vi "export.vi"(9 "Ruta luz":path, 10 "Ruta Temp":path, 11 "Curva de Luz y Temperatura 3":cluster{"Ramp Pattern":dbl[], u32[]}[](graph)=[{"Ramp Pattern"=[0.0, 0.25, 0.5, 0.75, 1.0, 1.25, 1.5, 1.75, 2.0, 2.25, 2.5, 2.75, 3.0, 3.25, 3.5, 3.75, 4.0, 4.25, 4.5, 4.75, 5.0, 5.25, 5.5, 5.75, 6.0, 6.25, 6.5, 6.75, 7.0, 7.25, 7.5, 7.75, 8.0, 8.25, 8.5, 8.75, 9.0, 9.25, 9.5, 9.75, 10.0, 10.25, 10.5, 10.75, 11.0, 11.25, 11.5, 11.75, 12.0, 12.25, 12.5, 12.75, 13.0, 13.25, 13.5, 13.75, 14.0, 14.25, 14.5, 14.75, 15.0, 15.25, 15.5, 15.75, 16.0, 16.25, 16.5, 16.75, 17.0, 17.25, 17.5, 17.75, 18.0, 18.25, 18.5, 18.75, 19.0, 19.25, 19.5, 19.75, 20.0, 20.25, 20.5, 20.75, 21.0, 21.25, 21.5, 21.75, 22.0, 22.25, 22.5, 22.75, 23.0, 23.25, 23.5, 23.75, 24.0, 24.25, 24.5, 24.75, 25.0, 25.25, 25.5, 25.75, 26.0, 26.25, 26.5, 26.75, 27.0, 27.25, 27.5, 27.75, 28.0, 28.25, 28.5, 28.75, 29.0, 29.25, 29.5, 29.75, 30.0, 30.25, 30.5, 30.75, 31.0, 31.25, 31.5, 31.75, 32.0, 32.25, 32.5, 32.75, 33.0, 33.25, 33.5, 33.75, 34.0, 34.25, 34.5, 34.75, 35.0, 35.25, 35.5, 35.75, 36.0, 36.25, 36.5, 36.75, 37.0, 37.25, 37.5, 37.75, 38.0, 38.25, 38.5, 38.75, 39.0, 39.25, 39.5, 39.75, 40.0, 40.25, 40.5, 40.75, 41.0, 41.25, 41.5, 41.75, 42.0, 42.25, 42.5, 42.75, 43.0, 43.25, 43.5, 43.75, 44.0, 44.25, 44.5, 44.75, 45.0, 45.25, 45.5, 45.75, 46.0, 46.25, 46.5, 46.75, 47.0, 47.25, 47.5, 47.75, 48.0, 48.25, 48.5, 48.75, 49.0, 49.25, 49.5, 49.75, 50.0, 50.25, 50.5, 50.75, 51.0, 51.25, 51.5, 51.75, 52.0, 52.25, 52.5, 52.75, 53.0, 53.25, 53.5, 53.75, 54.0, 54.25, 54.5, 54.75, 55.0, 55.25, 55.5, 55.75, 56.0, 56.25, 56.5, 56.75, 57.0, 57.25, 57.5, 57.75, 58.0, 58.25, 58.5, 58.75, 59.0, 59.25, 59.5, 59.75, 60.0, 60.25, 60.5, 60.75, 61.0, 61.25, 61.5, 61.75, 62.0, 62.25, 62.5, 62.75, 63.0, 63.25, 63.5, 63.75, 64.0, 64.25, 64.5, 64.75, 65.0, 65.25, 65.5, 65.75, 66.0, 66.25, 66.5, 66.75, 67.0, 67.25, 67.5, 67.75, 68.0, 68.25, 68.5, 68.75, 69.0, 69.25, 69.5, 69.75, 70.0, 70.25, 70.5, 70.75, 71.0, 71.25, 71.5, 71.75, 72.0, 72.25, 72.5, 72.75, 73.0, 73.25, 73.5, 73.75, 74.0, 74.25, 74.5, 74.75, 75.0, 75.25, 75.5, 75.75, 76.0, 76.25, 76.5, 76.75, 77.0, 77.25, 77.5, 77.75, 78.0, 78.25, 78.5, 78.75, 79.0, 79.25, 79.5, 79.75, 80.0, 80.25, 80.5, 80.75, 81.0, 81.25, 81.5, 81.75, 82.0, 82.25, 82.5, 82.75, 83.0, 83.25, 83.5, 83.75, 84.0, 84.25, 84.5, 84.75, 85.0, 85.25, 85.5, 85.75, 86.0, 86.25, 86.5, 86.75, 87.0, 87.25, 87.5, 87.75, 88.0, 88.25, 88.5, 88.75, 89.0, 89.25, 89.5, 89.75, 90.0, 90.25, 90.5, 90.75, 91.0, 91.25, 91.5, 91.75, 92.0, 92.25, 92.5, 92.75, 93.0, 93.25, 93.5, 93.75, 94.0, 94.25, 94.5, 94.75, 95.0, 95.25, 95.5, 95.75, 96.0, 96.25, 96.5, 96.75, 97.0, 97.25, 97.5, 97.75, 98.0, 98.25, 98.5, 98.75, 99.0, 99.25, 99.5, 99.75, 100.0, 100.25, 100.5, 100.75, 101.0, 101.25, 101.5, 101.75, 102.0, 102.25, 102.5, 102.75, 103.0, 103.25, 103.5, 103.75, 104.0, 104.25, 104.5, 104.75, 105.0, 105.25, 105.5, 105.75, 106.0, 106.25, 106.5, 106.75, 107.0, 107.25, 107.5, 107.75, 108.0, 108.25, 108.5, 108.75, 109.0, 109.25, 109.5, 109.75, 110.0, 110.25, 110.5, 110.75, 111.0, 111.25, 111.5, 111.75, 112.0, 112.25, 112.5, 112.75, 113.0, 113.25, 113.5, 113.75, 114.0, 114.25, 114.5, 114.75, 115.0, 115.25, 115.5, 115.75, 116.0, 116.25, 116.5, 116.75, 117.0, 117.25, 117.5, 117.75, 118.0, 118.25, 118.5, 118.75, 119.0, 119.25, 119.5, 119.75, 120.0, 120.25, 120.5, 120.75, 121.0], [36, 52, 52, 59, 71, 78, 91, 101, 109, 116, 119, 134, 137, 150, 160, 164, 175, 177, 190, 194, 199, 208, 218, 218, 229, 228, 234, 242, 250, 250, 261, 265, 270, 273, 278, 279, 307, 290, 296, 297, 306, 310, 311, 311, 317, 324, 324, 321, 339, 328, 339, 339, 342, 341, 343, 346, 343, 349, 350, 350, 350, 350, 350, 350, 350, 350, 350, 350, 350, 350, 350, 350, 350, 350, 350, 350, 350, 350, 350, 350, 350, 350, 350, 350, 350, 350, 350, 350, 350, 350, 350, 350, 350, 350, 350, 350, 350, 350, 350, 350, 350, 350, 350, 350, 350, 350, 350, 350, 350, 350, 350, 350, 350, 350, 350, 350, 350, 350, 350, 350, 0]}, ...(2 in all)]) -> ()   [LabVIEW 2021]
uses:
  <vilib>/Utility/file.llb/Write Delimited Spreadsheet (DBL).vi
panel:
  out "error out 2":errorcluster
  out "error out":errorcluster
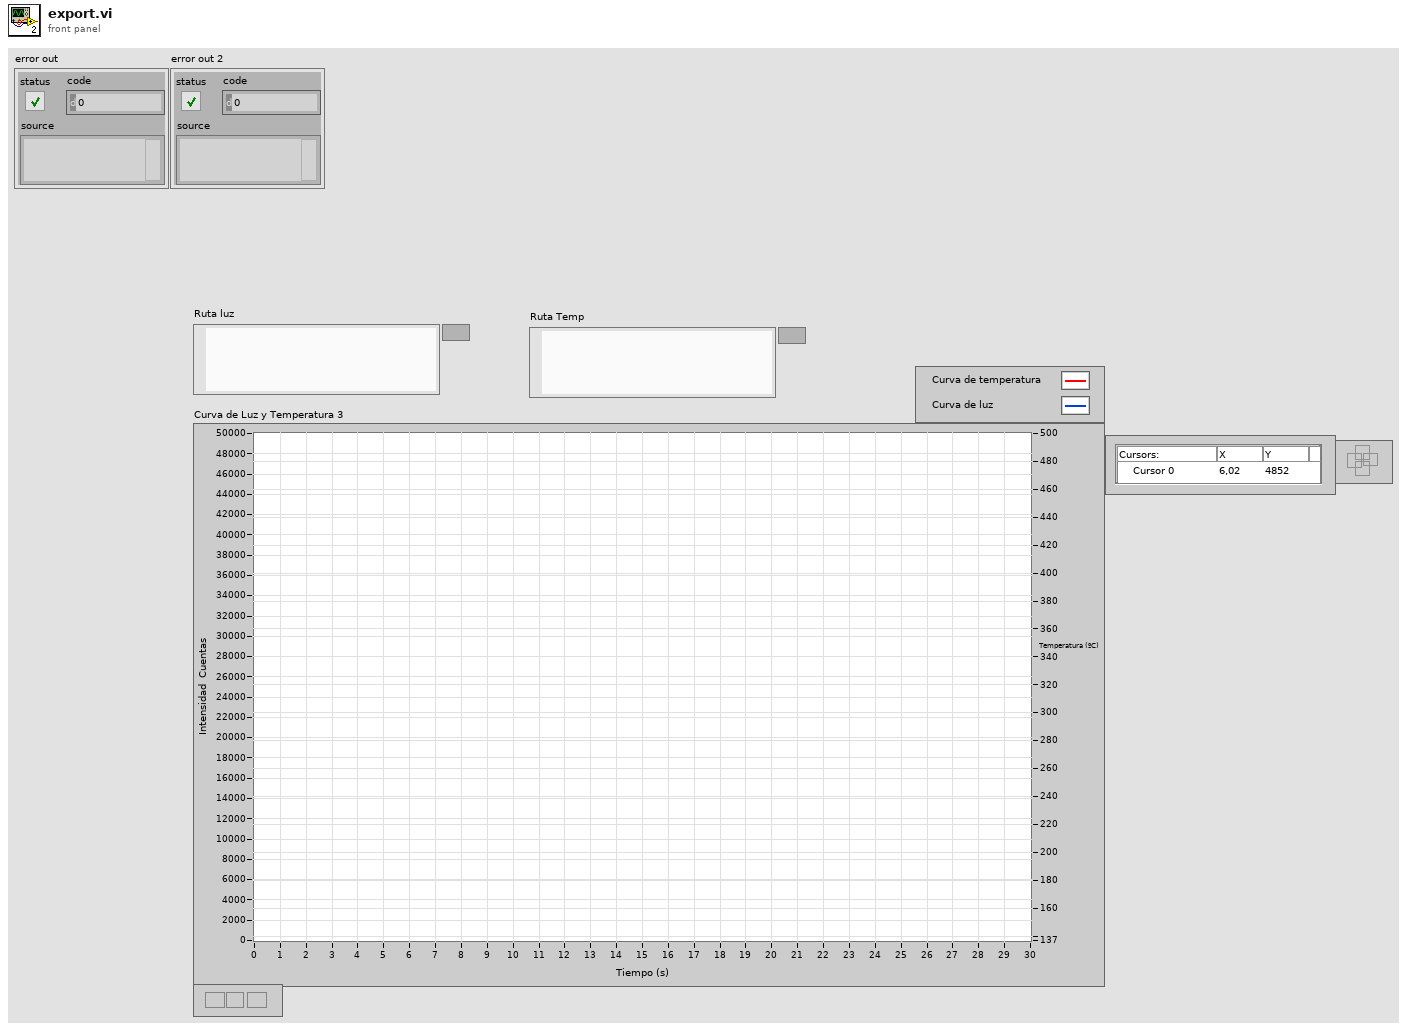
[diagram p1: front panel]
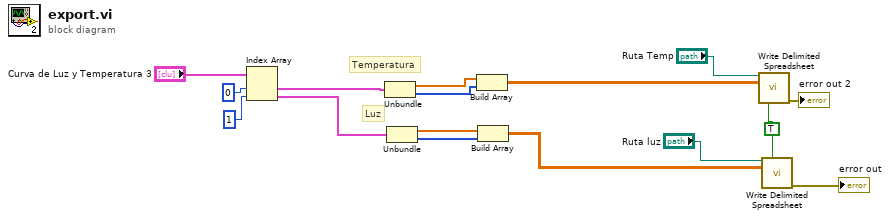
[diagram p0: block diagram]
diagram:
  w5 = TRUE ("transpose? (no:F)")
  # "Luz"
  # "Temperatura"
  n1 = Index Array(array="Curva de Luz y Temperatura 3", index #1=0 ("index"), index #2=1 ("index")) -> (element #1=w13:cluster{"Ramp Pattern":dbl[], u32[]}, element #2=w14:cluster{"Ramp Pattern":dbl[], u32[]})
  n2 = Unbundle(w13) -> ("Ramp Pattern"=w11:dbl[], w10:u32[])
  n3 = Unbundle(w14) -> ("Ramp Pattern"=w7:dbl[], w6:u32[])
  n4 = Build Array(w11, w10) -> (w8:dbl[][])
  n5 = Build Array(w7, w6) -> (w4:dbl[][])
  n6 = call-poly <vilib>:"Write Delimited Spreadsheet.vi"("file path (dialog if empty)"="Ruta Temp", "2D data"=w8, "transpose? (no:F)"=w5) -> ("error out"=→"error out 2":errorcluster)  [unwired: 11 in, 1 out]
  n7 = call-poly <vilib>:"Write Delimited Spreadsheet.vi"("file path (dialog if empty)"="Ruta luz", "2D data"=w4, "transpose? (no:F)"=w5) -> ("error out"=→"error out":errorcluster)  [unwired: 11 in, 1 out]
